vi "Test Base Card Passthrough (SLSC Switch).vi"() -> ()   [LabVIEW 2020, in "slsc-switch-benchmarks.lvlib"]
uses:
  slsc-switch-benchmarks.lvlib
panel:
  out "Array":dbl[](array[numeric])
  in  "Channels to Sweep":i32=64
  out "#Channels Testing":i32
  out "Avg Connection Time":dbl(graph)
  in  "device":refnum<k21>="SET-2010-Mod2"
  in  "Disconnection":T1(ring)=enum."Disconnect Single"
  in  "Connection":enum16{"Connect Single", "Connect Array"}(ring)=enum."Connect Array"
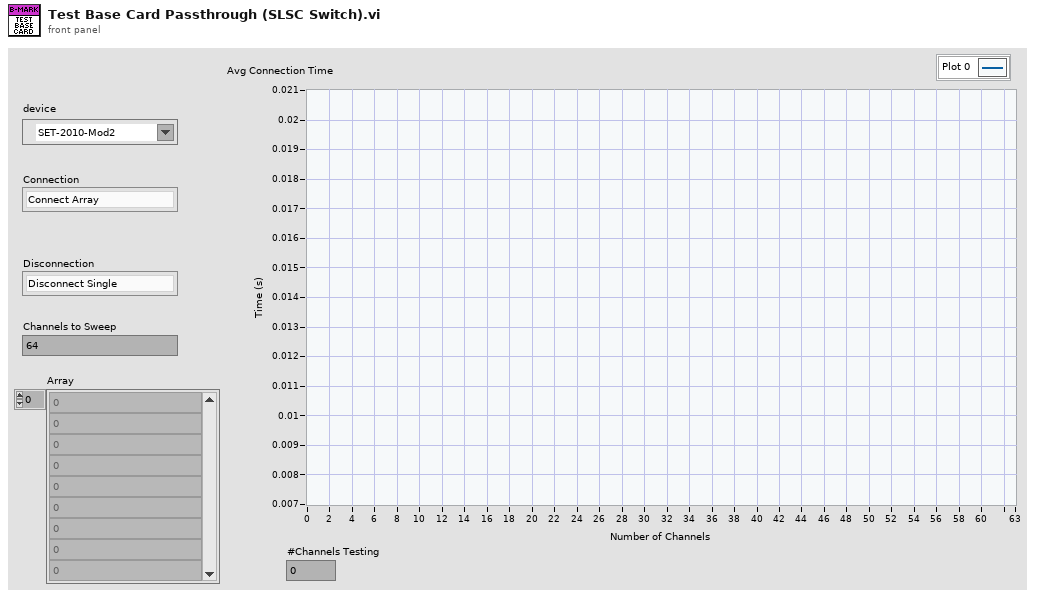
[diagram p1: front panel]
types:
  T1 = enum16{"No-Op", "Disconnect Single", "Disconnect Array", "Disconnect All"}
  T2 = typedef "slsc-switch-benchmarks.lvlib/Timing Statistics.ctl" = cluster{"mean":dbl, "standard deviation":dbl, "maximum time":dbl, "minimum time":dbl}
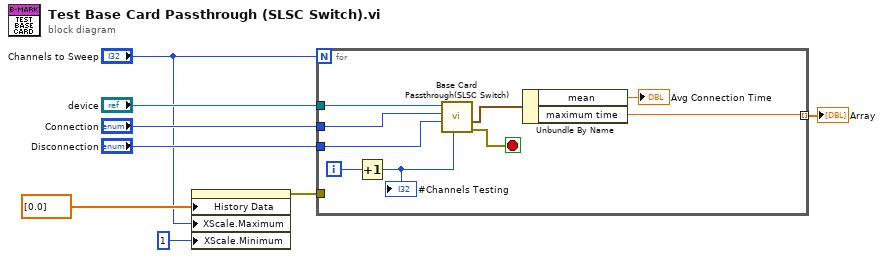
[diagram p0: block diagram]
diagram:
  n1 = property on="Avg Connection Time" class="WFChart (strict)"("History Data"=dbl[] [0.0], "XScale.Maximum"="Channels to Sweep", "XScale.Minimum"=1 ("Channels to Sweep")) -> (error out=w4:errorcluster)  [unwired: 2 in, 1 out]
  n2 = for {
    N: "Channels to Sweep" -> [_]
    tunnel: "Connection" -> [w15]
    tunnel: "Disconnection" -> [w14]
    tunnel: "device" -> [w13]
    tunnel: w4 -> [_]
    tunnel: [w10] -> w3 mode=indexing
    i -> [w17]
    stop <- w12 stop-if-true
    n3 = Increment(x=w17) -> (x+1=w16:i32)
    "#Channels Testing" <- w16
    n4 = call "Base Card Passthrough(SLSC Switch).vi"("Channels (1-64)"=w16, "Disconnection"=w14, "Connection"=w15, "device"=w13) -> ("error out"=w12:errorcluster, "Disconnect Timing"=w9:T2)  [unwired: 5 in, 1 out]
    n5 = Unbundle By Name(w9) -> ("mean"=→"Avg Connection Time":dbl, "maximum time"=w10:dbl)
  }
  "Array" <- w3
